vi "IP Resolver.vi"(8 "error in (no error)":errorcluster, 11 "Node Config in":refnum<class "Node Config.lvclass">) -> (0 "error out":errorcluster, 2 "IP Resolver":refnum<class "IP Resolver.lvclass">, 3 "Node Config out":refnum<class "Node Config.lvclass">)   [LabVIEW 2020, in "VectoConfig.lvlib" / "Node Config.lvclass"]
uses:
  Node Config.lvclass
  Node Config.lvclass/Node Config.ctl
  IP Resolver/IP Resolver.lvclass
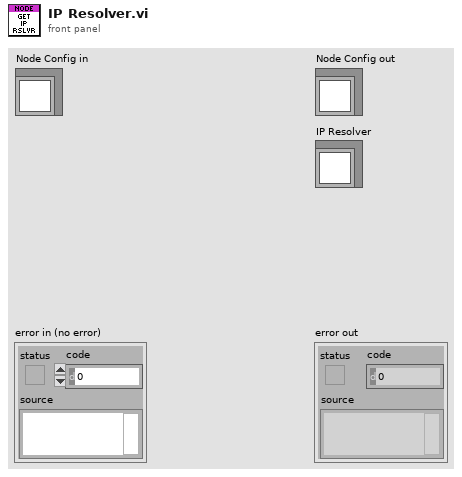
[diagram p1: front panel]
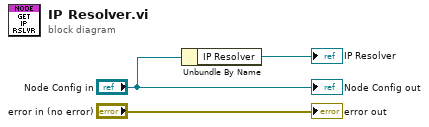
[diagram p0: block diagram]
diagram:
  n1 = Unbundle By Name("Node Config in") -> ("IP Resolver"=→"IP Resolver":refnum<class "IP Resolver.lvclass">)
  "error out" <- "error in (no error)"
  "Node Config out" <- "Node Config in"
